vi "CMD_FAT_GENERIC_Command_ACK.vi"(0 "Input_Data":string[](array[string]), 5 "Error In":errorcluster) -> (12 "Validate CheckSum":bool, 13 "Command":u8[](array[numeric])=[4, 228, 4, 128, 0, 0, 0, 0, 0, 0, 0, 0, 0, 0] format="%x", 14 "Response":bool, 15 "Ack":bool, 16 "Command":bool, 17 "Add CheckSum":bool, 18 "Status":bool, 19 "Error Out":errorcluster)   [LabVIEW 2014]
panel:
  out "Array":u8[](array[numeric]) format="%x"
  # "Flags"
  # "FAT_Generic Command:"
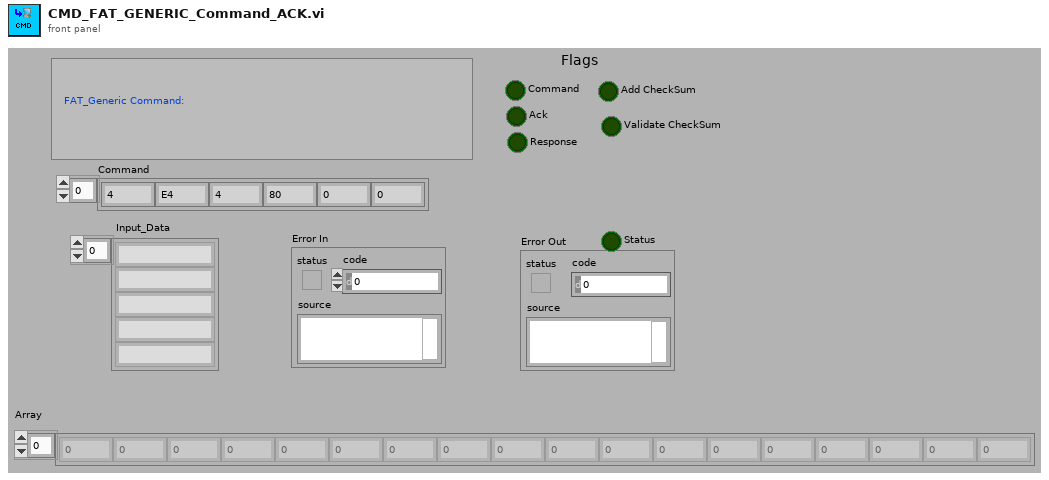
[diagram p1: front panel]
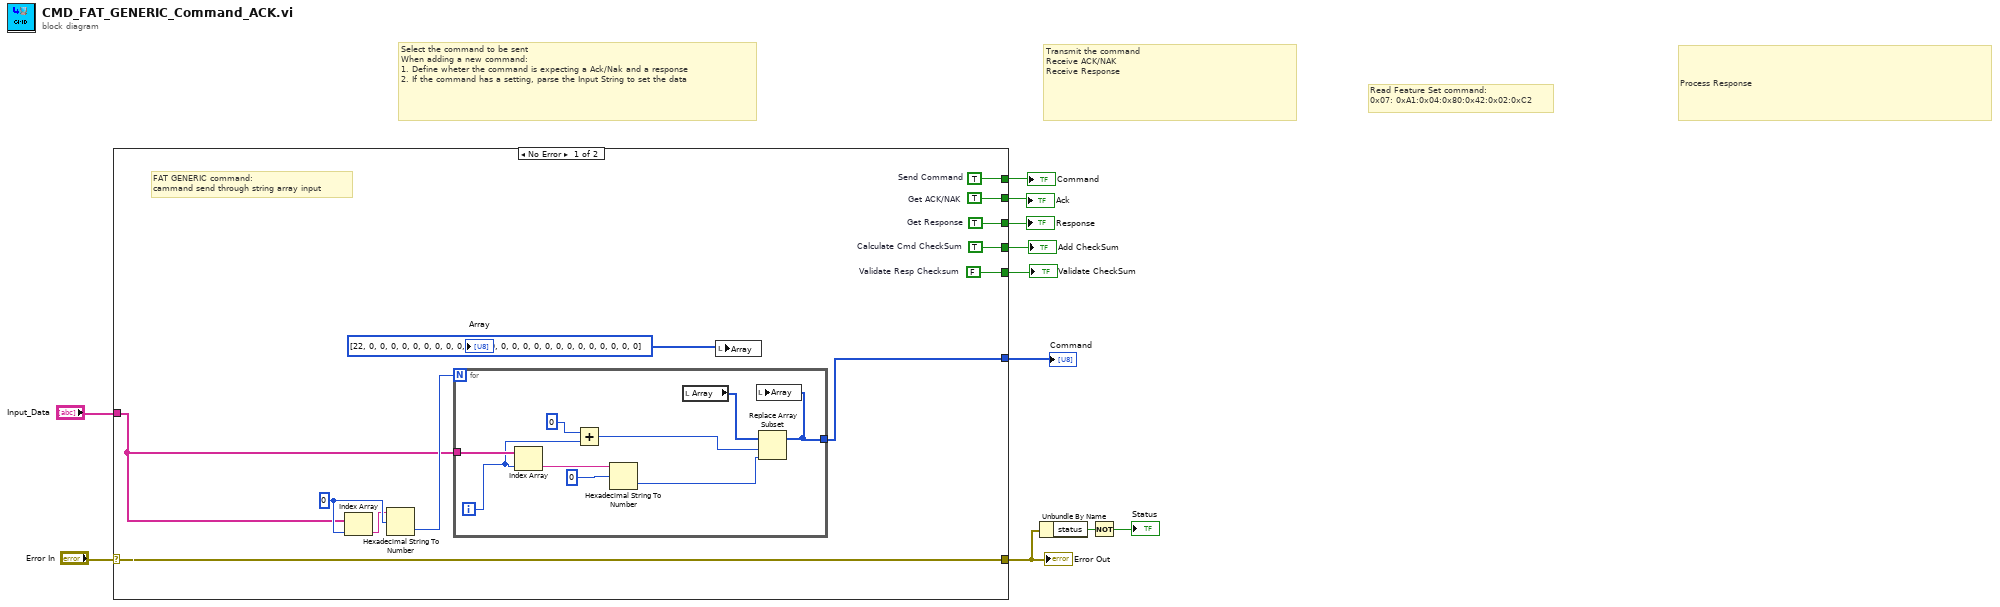
[diagram p0: block diagram]
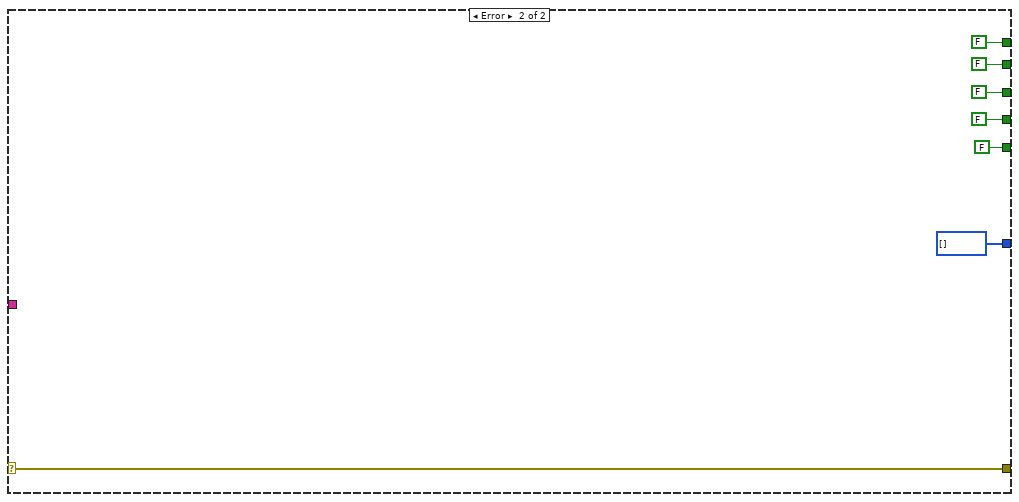
[diagram p2: hidden frame]
diagram:
  # "Read Feature Set command:\n0x07: 0xA1:0x04:0x80:0x42:0x02:0xC2"
  # "Process Response"
  # "Transmit the command\nReceive ACK/NAK\nReceive Response"
  # "Select the command to be sent\nWhen adding a new command:\n1. Define wheter the command is expecting a Ack/Nak and a response\n2. If the command has a setting, parse the Input String to set the data"
  n1 = case shown="No Error" "Error In" {
    selector: "Error In" -> [w19 w34]
    tunnel: [w23 FALSE ("Send Command")] -> w10
    tunnel: [w22 FALSE ("Get ACK/NAK")] -> w9
    tunnel: [w21 FALSE ("Get Response")] -> w8
    tunnel: [w20 FALSE ("Add CheckSum")] -> w7
    tunnel: [w12 u8[] []] -> w6
    tunnel: [w19 w34] -> w4
    tunnel: "Input_Data" -> [w13 _]
    tunnel: [w18 FALSE ("Validate Resp Checksum")] -> w1
    frame No Error {
      w16 = 0 ("offset")
      w18 = FALSE  # Validate Resp Checksum
      w20 = TRUE  # Calculate Cmd CheckSum
      w21 = TRUE  # Get Response
      w23 = TRUE  # Send Command
      w22 = TRUE  # Get ACK/NAK
      # "FAT GENERIC command:\ncammand send through string array input"
      n2 = Index Array(array=w13, index=w16) -> (element=w15:string)
      n3 = Hexadecimal String To Number(string=w15, offset=w16) -> (number=w14:u32)  [unwired: 1 in, 1 out]
      n4 = for {
        N: w14 -> [_]
        tunnel: w13 -> [w32]
        tunnel: [w27] -> w12
        i -> [w29]
        n5 = Index Array(array=w32, index=w29) -> (element=w26:string)
        n6 = Add(x=0 ("index"), y=w29) -> (x+y=w30:i32)
        n7 = Hexadecimal String To Number(string=w26, offset=0) -> (number=w24:u32)  [unwired: 1 in, 1 out]
        n8 = local read "Array"() -> (w28:u8[])
        n9 = Replace Array Subset(array=w28, new element=w24, index=w30) -> (w27:u8[])
        n10 = local write "Array"(w27) -> ()
      }
      n11 = local write "Array"(u8[] [22, 0, 0, 0, 0, 0, 0, 0, 0, 0, 0, 0, 0, 0, 0, 0, 0, 0, 0, 0, 0, 0, 0, 0, 0, 0]) -> ()
    }
    frame Error {
    }
  }
  "Error Out" <- w4
  "Command" <- w10
  "Ack" <- w9
  "Response" <- w8
  "Add CheckSum" <- w7
  "Command" <- w6
  "Validate CheckSum" <- w1
  n12 = Unbundle By Name(w4) -> ("status"=w3:bool)
  n13 = Not(x=w3) -> (.not. x?=→"Status":bool)
